vi "set Front Panel Resizable.vi"(8 "error in (no error)":errorcluster, 10 "Front Panel Resizable":bool, 11 "Actor in":refnum<class "Actor.lvclass">) -> (0 "error out":errorcluster, 3 "Actor out":refnum<class "Actor.lvclass">)   [LabVIEW 2015, in "Actor.lvclass"]
uses:
  Actor.lvclass
  Actor.lvclass/Actor.ctl
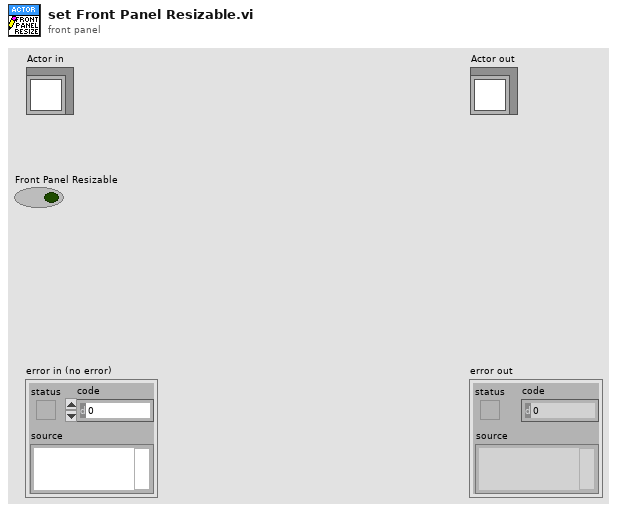
[diagram p1: front panel]
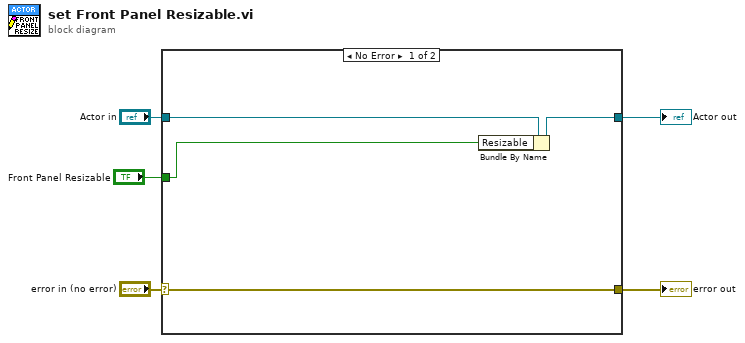
[diagram p0: block diagram]
diagram:
  n1 = case shown="No Error" "error in (no error)" {
    selector: "error in (no error)" -> [w6 w10]
    tunnel: [w6 w10] -> w4
    tunnel: [w9 w11] -> w2
    tunnel: "Actor in" -> [w8 w11]
    tunnel: "Front Panel Resizable" -> [w7 _]
    frame No Error {
      n2 = Bundle By Name(cluster=w8, "Resizable"=w7) -> (w9:refnum<class "Actor.lvclass">)
    }
    frame Error {
    }
  }
  "error out" <- w4
  "Actor out" <- w2
